vi "player-test.vi"() -> ()   [LabVIEW 2012]
uses:
  player_glo.vi
  musicplayer_glo.vi
  test_glo.vi
panel:
  out "error-playstate":errorcluster
  out "error out":errorcluster caption="Fehler (Ausgang)"
  out "running?":bool
  in  "stop-vi":bool
  out "playing?":bool
  out "playState":i32(ring) items=["wmppsUndefined", "wmppsStopped", "wmppsPaused", "wmppsPlaying", "wmppsScanForward", "wmppsScanReverse", "wmppsBuffering", "wmppsWaiting", "wmppsMediaEnded", "wmppsTransitioning", "wmppsReady", "wmppsReconnecting", "wmppsLast"]
  out "error-pool":errorcluster caption="Fehler (Ausgang)"
  out "playerkernel referenz":refnum<vi>
  in  "stop":bool
  out "Log":string
  in  "play":bool
  in  "Pfad":path
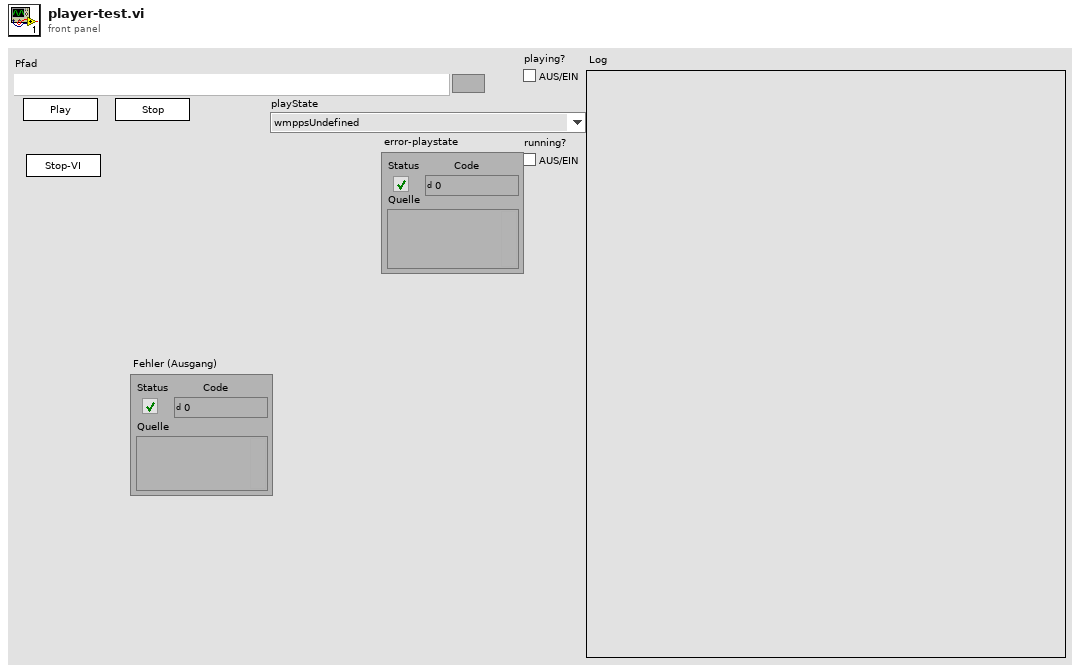
[diagram p1: front panel]
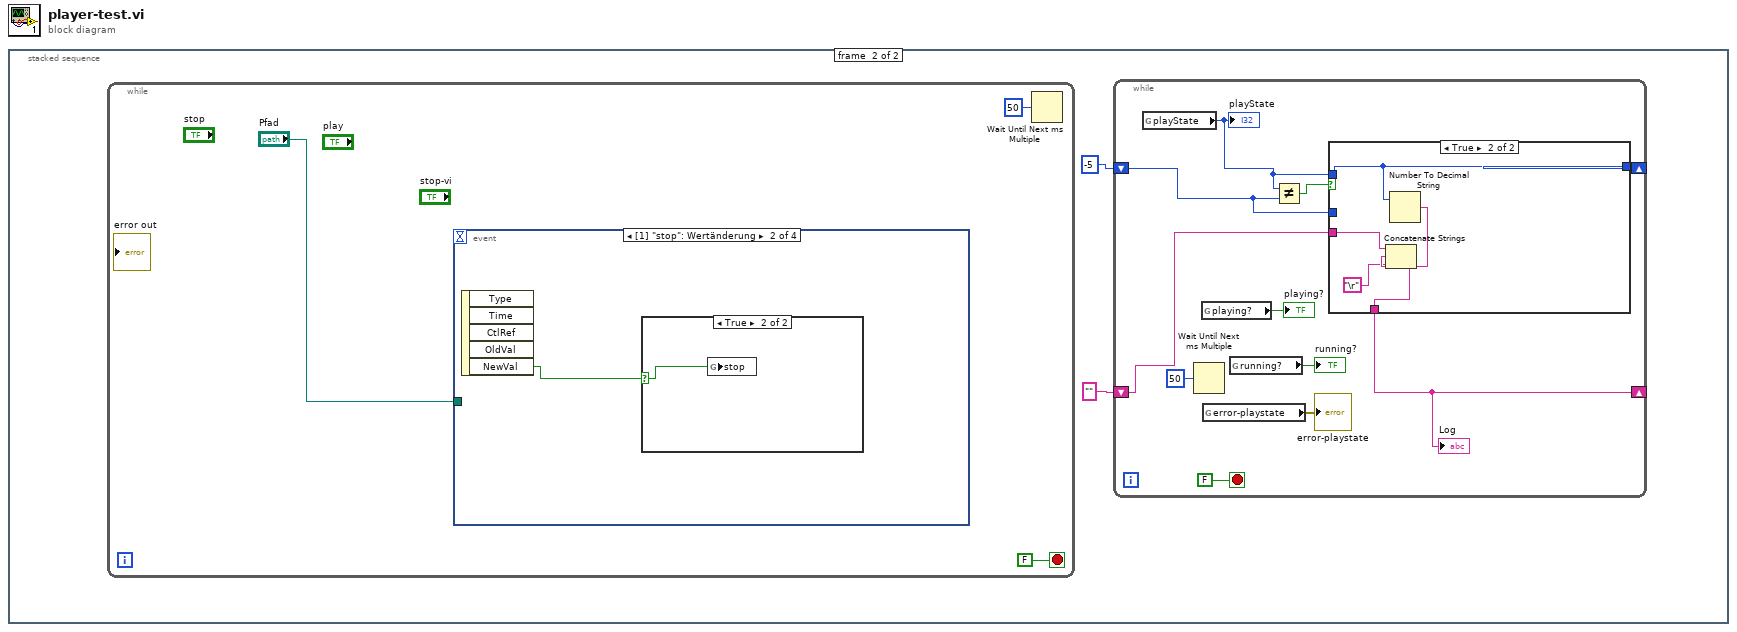
[diagram p0: block diagram]
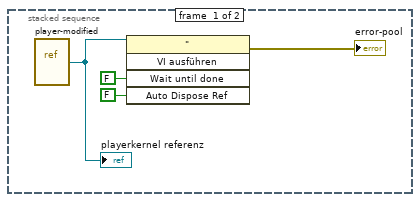
[diagram p2: hidden frame]
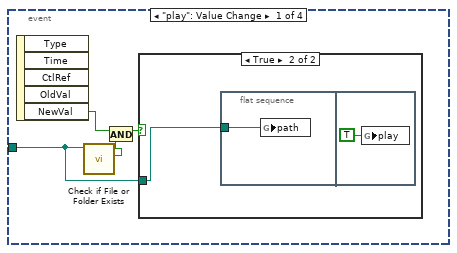
[diagram p4: hidden frame]
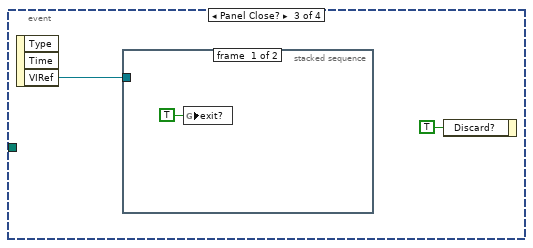
[diagram p7: hidden frame]
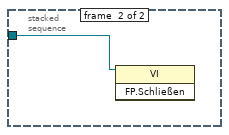
[diagram p8: hidden frame]
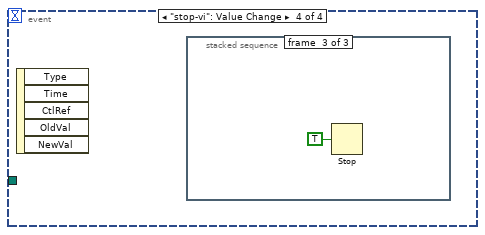
[diagram p9: hidden frame]
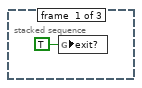
[diagram p10: hidden frame]
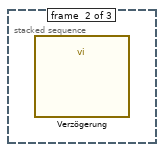
[diagram p11: hidden frame]
diagram:
  n1 = stacked-sequence {
    frame #0 {
      n2 = vi-ref "player-modified.vi"() -> (w2:refnum<vi>)
      "playerkernel referenz" <- w2
      n3 = invoke class="\"" method="VI ausführen"(reference=w2, "Wait until done"=FALSE ("Warten bis beendet"), "Auto Dispose Ref"=FALSE ("Referenz automatisch schließen")) -> (error out=→"error-pool":errorcluster)  [unwired: 2 in, 4 out]
    }
    frame #1 {
      n4 = while {
        stop <- FALSE stop-if-true
        n5 = event shown="[1] \"stop\": Wertänderung" {
          selector: _ -> [_ _ _ _]
          dyn-events: _ -> [_ _ _ _]
          timeout: _ -> [_ _ _ _]
          tunnel: "Pfad" -> [w28 _ _ _]
          event "play": Value Change {
            n6 = event-data() -> ("NewVal"=w31:bool)  [unwired: 1 in, 4 out]
            n7 = call <vilib>:"Check if File or Folder Exists.vi"("path"=w28) -> ("file or folder exists?"=w29:bool)  [unwired: 8 in, 2 out]
            n8 = And(x=w31, y=w29) -> (x .and. y?=w30:bool)
            n9 = case shown="True" w30 {
              tunnel: w28 -> [_ w32]
              frame False {
              }
              frame True {
                n10 = flat-sequence {
                  tunnel: w32 -> [w33]
                  frame #0 {
                    n11 = global write "player_glo.vi" "path"(w33) -> ()
                  }
                  frame #1 {
                    n12 = global write "player_glo.vi" "play"(TRUE ("play")) -> ()
                  }
                }
              }
            }
          }
          event "stop": Value Change {
            n13 = event-data() -> ("NewVal"=w35:bool)  [unwired: 1 in, 4 out]
            n14 = case shown="True" w35 {
              selector: w35 -> [_ w36]
              frame False {
              }
              frame True {
                n15 = global write "player_glo.vi" "stop"(w36) -> ()
              }
            }
          }
          event Panel Close? {
            n16 = event-data() -> ("VIRef"=w37:refnum<vi>)  [unwired: 1 in, 2 out]
            n17 = stacked-sequence {
              tunnel: w37 -> [_ w40]
              frame #0 {
                n18 = global write "musicplayer_glo.vi" "exit?"(TRUE ("exit?")) -> ()
              }
              frame #1 {
                n19 = invoke class="VI" method="FP.Schließen"(reference=w40) -> ()  [unwired: 2 in, 3 out]
              }
            }
            n20 = event-data("Discard?"=TRUE ("Verwerfen?")) -> ()  [unwired: 1 in, 1 out]
          }
          event "stop-vi": Value Change {
            n21 = event-data() -> ()  [unwired: 1 in, 5 out]
            n22 = stacked-sequence {
              frame #0 {
                n23 = global write "musicplayer_glo.vi" "exit?"(TRUE ("exit?")) -> ()
              }
              frame #1 {
                n24 = call "Verzögerung"() -> ()  [unwired: 11 in, 1 out]
              }
              frame #2 {
                n25 = Stop(stop? (T)=TRUE ("Stopp? (T)")) -> ()
              }
            }
          }
        }
        n26 = Wait Until Next ms Multiple(millisecond multiple=u32 50 ("Vielfache von ms")) -> ()  [unwired: 1 out]
      }
      n27 = while {
        shift-right: [w12] -> _
        shift-left: -5 -> [w10]
        shift-right: [w8] -> _
        shift-left: "" -> [w9]
        stop <- FALSE stop-if-true
        n28 = global read "player_glo.vi" "playState"() -> (w11:i32)
        "playState" <- w11
        n29 = Wait Until Next ms Multiple(millisecond multiple=u32 50 ("Vielfache von ms")) -> ()  [unwired: 1 out]
        n30 = global read "musicplayer_glo.vi" "playing?"() -> (→"playing?":bool)
        n31 = global read "test_glo.vi" "error-playstate"() -> (→"error-playstate":errorcluster)
        n32 = global read "player_glo.vi" "running?"() -> (→"running?":bool)
        n33 = Not Equal?(x=w11, y=w10) -> (x != y?=w13:bool)
        n34 = case shown="True" w13 {
          tunnel: [w19 w23] -> w12
          tunnel: w11 -> [_ w23]
          tunnel: w10 -> [w19 _]
          tunnel: [w18 w20] -> w8
          tunnel: w9 -> [w18 w24]
          frame False {
          }
          frame True {
            n35 = Number To Decimal String(number=w23) -> (decimal integer string=w22:string)  [unwired: 1 in]
            n36 = Concatenate Strings(w24, w22, "\r") -> (w20:string)
          }
        }
        "Log" <- w8
      }
    }
  }
